vi "ReglerSubVI.vi"(0 "Queue Reference":refnum<queue>, 11 "Error IN":errorcluster) -> (15 "error OUT":errorcluster)   [LabVIEW 2016]
uses:
  <vilib>/Simulation/Scripting/Companion Diagram/SimConfigNode/SimParams.ctl
  <vilib>/Simulation/Scripting/Companion Diagram/SimConfigNode/_simSolvers.ctl
  <vilib>/Simulation/Implementation/Shared/SIMSCR Execution Mode.ctl
  <vilib>/Platform/TimedLoop/XDataNode/timing_clust.ctl
  <vilib>/Platform/TimedLoop/XDataNode/nitl_modes.ctl
  <vilib>/Platform/TimedLoop/XDataNode/wakeup.ctl
  <vilib>/Simulation/Param Hierarchy/Typedefs/SIMPH Param Control Actions.ctl
  <vilib>/Simulation/Implementation/Shared/SIM limit type.ctl
  <vilib>/Simulation/Scripting/Editor Utilities/SIM subVI tag data.ctl
  <vilib>/Simulation/Scripting/Editor Utilities/SIM subVI execution type.ctl
  <vilib>/Simulation/Implementation/Shared/NILVSim_ParamChanged.vi
  <vilib>/Simulation/Implementation/Shared/NILVSim_FinishedLate.vi
  <vilib>/Simulation/Implementation/Shared/NILVSIM_BeginStep.vi
  <vilib>/Simulation/Utility/Implementation/SIM Halt.vi
  <vilib>/Simulation/SignalArithmetic/Implementation/NILVSim Gain.llb/SIM Gain (scalar).vi
  <vilib>/Simulation/ContinuousLinear/Implementation/NILVSim Derivative.llb/SIM derivative (scalar).vi
  <vilib>/Simulation/Nonlinear/Implementation/NILVSim Saturation.llb/SIM Saturation (scalar).vi
  <vilib>/Simulation/ContinuousLinear/Implementation/NILVSim Integrator new.llb/SIM Integrator distributor (scalar).vi
  <vilib>/Simulation/ContinuousLinear/Implementation/NILVSim Integrator new.llb/SIM Integrator collector (scalar).vi
  <vilib>/Simulation/Implementation/Shared/SIM Fire Discrete SubVI.vi
  <vilib>/Simulation/Implementation/Shared/NILVSim_Manager.vi
  <vilib>/Utility/error.llb/Clear Errors.vi
  <vilib>/Simulation/Implementation/Shared/NILVSim_FinalizeModel.vi
  <vilib>/Simulation/Implementation/Shared/SIM Fire Discrete SubVI (Core).vi
  <vilib>/Simulation/Implementation/Shared/SIM Unbundle Sim Info.vi
  <vilib>/Simulation/Implementation/Shared/SIMSH Read Queue.vi
  Globale Variablen VI/AutonomousMode.vi
  Globale Variablen VI/Global Variables.vi
  Globale Variablen VI/RadSensoren.vi
  <vilib>/Simulation/Implementation/Shared/NILVSim_Initialize.vi
  <vilib>/Simulation/Utility/Implementation/NILVSim Get Time and IsAcceptedStep.vi
  Globale Variablen VI/Logging Globale Variable.vi
  <vilib>/Simulation/Implementation/Shared/NILVSim_GetModelError.vi
  <vilib>/Simulation/Implementation/Shared/SIM Bundle Sim Info.vi
  <vilib>/Simulation/Scripting/Companion Diagram/SimConfigNode/SimDog.xnode
  <vilib>/Platform/TimedLoop/XDataNode/XDataNode.xnode
  <vilib>/Simulation/Implementation/XNodeFramework/SimXNode/SimX.xnode
  <vilib>/Simulation/ContinuousLinear/Implementation/NILVSim Integrator new.llb/SIM Integrator (scalar).vi
  <vilib>/Platform/TimedLoop/XDataNode/XDNodeRunTimeDep.lvlib
  <vilib>/Simulation/Implementation/Shared/NI_SIM_Implementation.lvlib
panel:
  out "vs":dbl
  out "throttle voltage":dbl(knob) scale=0.4..5.0
  out "brake voltage":dbl(knob) scale=0.0..12.0
  out "velocity (m/s)":dbl(knob) scale=0.0..50.0
  # "V3"
  # "Hebebühne:\nb_kp: 1\nb_Ti: 0\nb_Td: 0"
  # "Strasse:\nb_kp: 1.5 \nb_Ti: 0\nb_Td: 0"
  # "Hebebühne:\nt_kp: 1.5\nt_Ti: 0.1\nt_Td: 0"
  # "Strasse:\nt_kp: 2.5 \nt_Ti: 0.3 \nt_Td: 0"
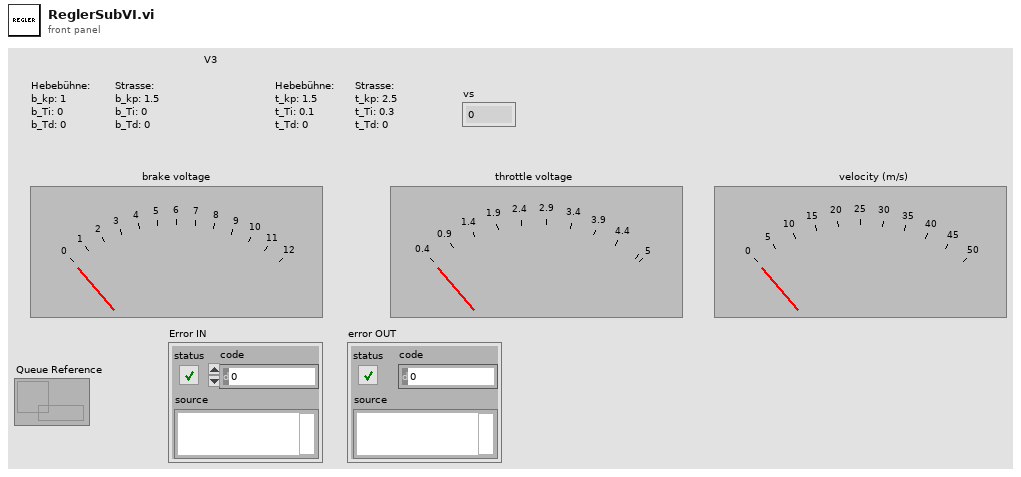
[diagram p1: front panel]
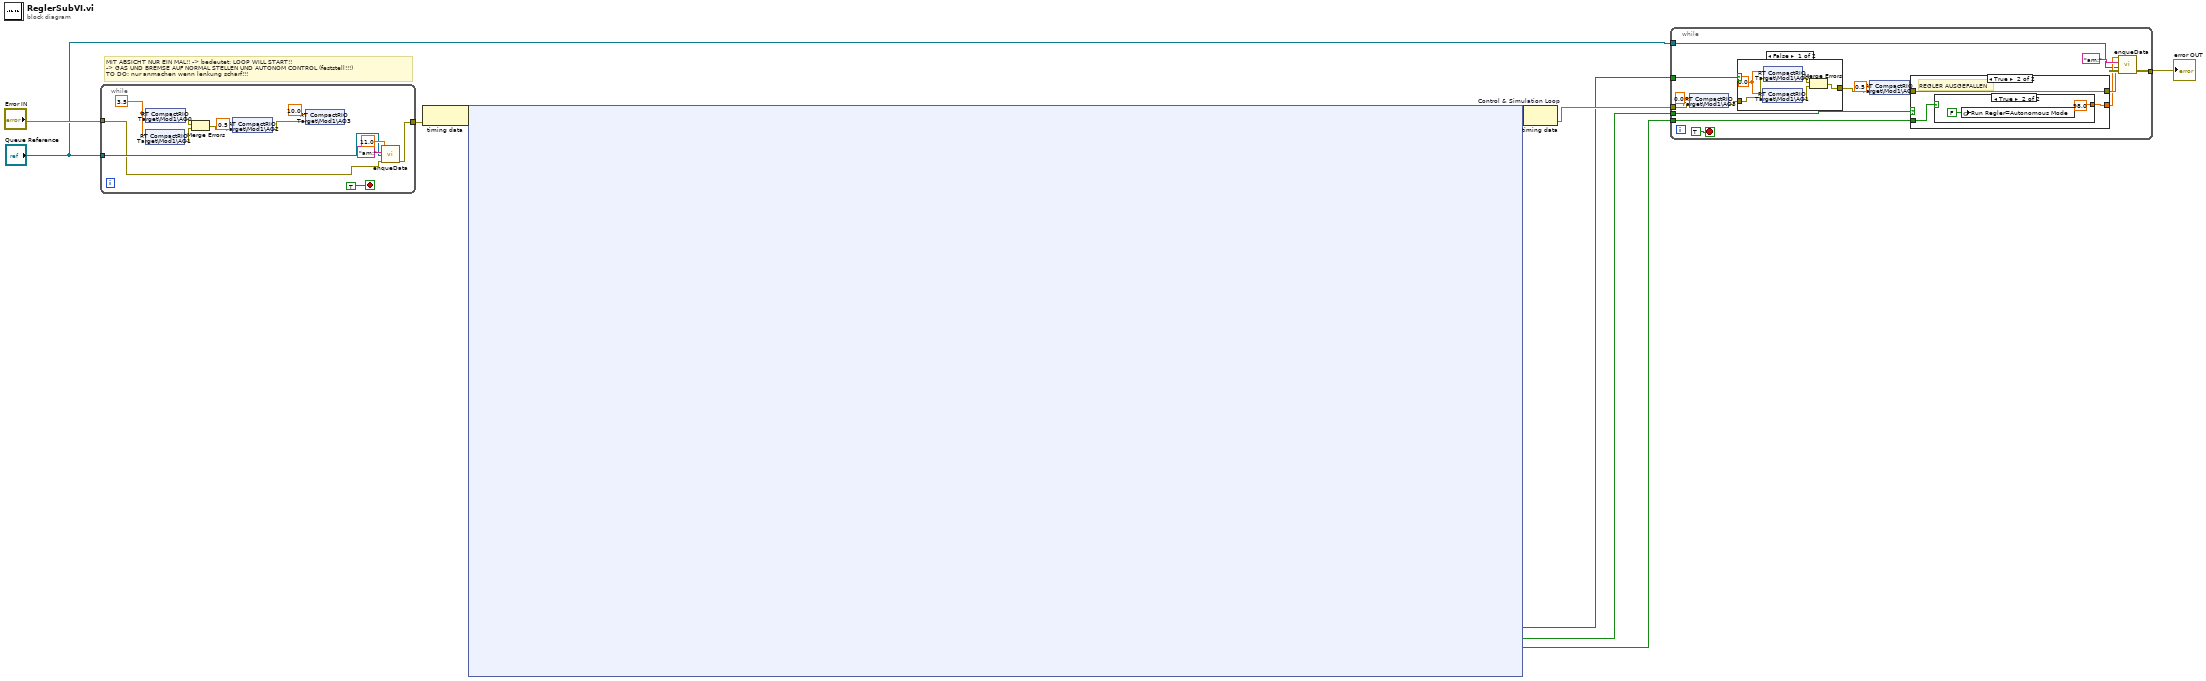
[diagram p0: block diagram]
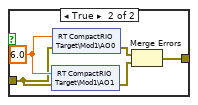
[diagram p2: hidden frame]
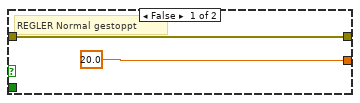
[diagram p3: hidden frame]
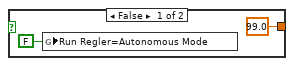
[diagram p4: hidden frame]
diagram:
  # "MIT ABSICHT NUR EIN MAL!! -> bedeutet: LOOP WILL START!! \n-> GAS UND BREMSE AUF NORMAL STELLEN UND AUTONOM CONTROL (feststell!!!)\nTO DO: nur anmachen wenn lenkung scharf!!!"
  n1 = while {
    tunnel: "Error IN" -> [w11]
    tunnel: [w19] -> w8
    tunnel: "Queue Reference" -> [w12]
    stop <- TRUE stop-if-true
    w14 = 3.5
    n2 = shared-variable "RT CompactRIO Target\\Mod1\\AO1"(w14) -> (error out=w16:errorcluster)  [unwired: 1 in]
    n3 = shared-variable "RT CompactRIO Target\\Mod1\\AO0"(w14) -> (error out=w17:errorcluster)  [unwired: 1 in]
    n4 = Merge Errors(w17, w16) -> (w18:errorcluster)
    n5 = shared-variable "RT CompactRIO Target\\Mod1\\AO2"(0.5, error in=w18) -> (error out=w13:errorcluster)
    n6 = shared-variable "RT CompactRIO Target\\Mod1\\AO3"(10.0 ("t 2"), error in=w13) -> ()  [unwired: 1 out]
    n7 = call "enqueData.vi"("error in (no error)"=w11, "Queue Reference"=w12, "Descriptor"="am:", "Value IN"=11.0) -> ("error out"=w19:errorcluster)  [unwired: 7 in]
  }
  n8 = node-c288(w8) -> (w10:variant)
  n9 = node-c254 "Control & Simulation Loop"(w10) -> (w9:variant, w4:bool, w2:bool, w1:bool)
  n10 = node-c288(w9) -> (w5:errorcluster)
  n11 = while {
    tunnel: [w32] -> w3
    tunnel: w5 -> [w31]
    tunnel: w4 -> [w28]
    tunnel: "Queue Reference" -> [w26]
    tunnel: w2 -> [w25]
    tunnel: w1 -> [w24]
    stop <- TRUE stop-if-true
    n12 = shared-variable "RT CompactRIO Target\\Mod1\\AO3"(0.0 ("t 2"), error in=w31) -> (error out=w34:errorcluster)
    n13 = case shown="False" w24 {
      tunnel: w34 -> [w40 w47]
      tunnel: [w39 w44] -> w33
      frame False {
        w43 = 0.0
        n14 = shared-variable "RT CompactRIO Target\\Mod1\\AO1"(w43) -> (error out=w42:errorcluster)  [unwired: 1 in]
        n15 = shared-variable "RT CompactRIO Target\\Mod1\\AO0"(w43, error in=w40) -> (error out=w41:errorcluster)
        n16 = Merge Errors(w41, w42) -> (w39:errorcluster)
      }
      frame True {
        w48 = 6.0
        n17 = shared-variable "RT CompactRIO Target\\Mod1\\AO1"(w48, error in=w47) -> (error out=w46:errorcluster)
        n18 = shared-variable "RT CompactRIO Target\\Mod1\\AO0"(w48, error in=w47) -> (error out=w45:errorcluster)
        n19 = Merge Errors(w45, w46) -> (w44:errorcluster)
      }
    }
    n20 = shared-variable "RT CompactRIO Target\\Mod1\\AO2"(0.5, error in=w33) -> (error out=w30:errorcluster)
    n21 = case shown="True" w28 {
      tunnel: w30 -> [w50 w53]
      tunnel: [w50 w53] -> w29
      tunnel: [20.0 ("Value IN") w51] -> w27
      tunnel: w25 -> [_ w52]
      frame False {
        # "REGLER Normal gestoppt"
      }
      frame True {
        # "REGLER AUSGEFALLEN"
        n22 = case shown="True" w52 {
          tunnel: [99.0 ("Value IN") 98.0 ("Value IN")] -> w51
          frame False {
            n23 = global write "AutonomousMode.vi" "Run Regler=Autonomous Mode"(FALSE ("Run Regler=Autonomous Mode")) -> ()
          }
          frame True {
            n24 = global write "AutonomousMode.vi" "Run Regler=Autonomous Mode"(FALSE ("Run Regler=Autonomous Mode")) -> ()
          }
        }
      }
    }
    n25 = call "enqueData.vi"("error in (no error)"=w29, "Queue Reference"=w26, "Descriptor"="am:", "Value IN"=w27) -> ("error out"=w32:errorcluster)  [unwired: 7 in]
  }
  "error OUT" <- w3
